vi "RX-SIS-BPCS-Modbus (SubVI).vi"(8 "error in (no error)":errorcluster, 11 "Modbus Master in":refnum<class "Modbus Master.lvclass">) -> (0 "error out":errorcluster, 1 "SIS-10SDV501":bool, 2 "SIS-10SDV500":bool, 3 "Modbus Master out":refnum<class "Modbus Master.lvclass">, 5 "SIS-10SDV502":bool, 7 "SIS-BPCS-RX-Array":bool[](array[boolean]))   [LabVIEW 2018]
uses:
  <vilib>/Modbus/master/Modbus Master.lvclass
  BPCS Global Variables.vi
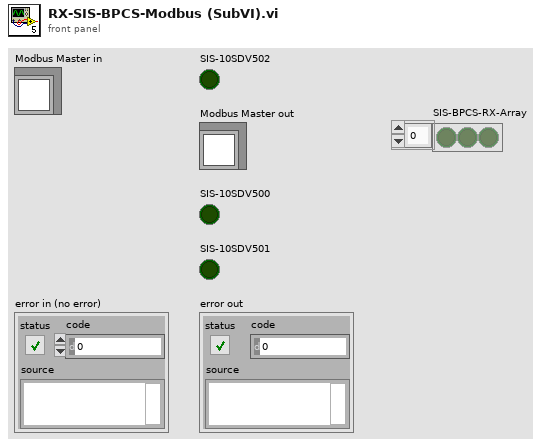
[diagram p1: front panel]
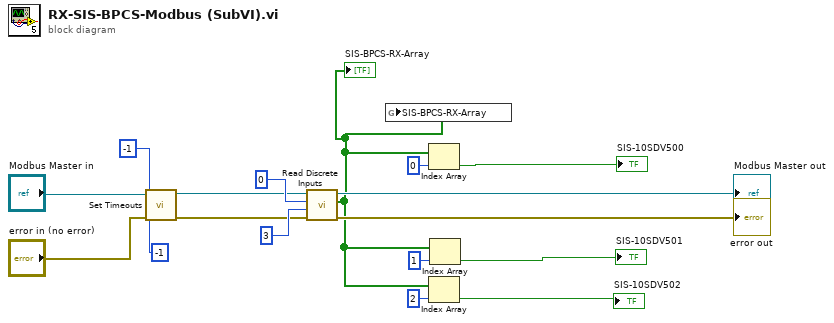
[diagram p0: block diagram]
diagram:
  n1 = call <vilib>:"Set Timeouts.vi"("error in (no error)"="error in (no error)", "write operation timeout (ms)"=-1, "read operation timeout (ms)"=-1, "Modbus master in"="Modbus Master in") -> ("error out"=w4:errorcluster, "Modbus master out"=w5:refnum<class "Modbus Master.lvclass">)  [unwired: 6 in]
  n2 = call-dynamic "Read Discrete Inputs.vi"("error in (no error)"=w4, "number of discrete inputs"=u16 3, "starting address"=u16 0, "Modbus master in"=w5) -> ("error out"=→"error out":errorcluster, "discrete input values"=w6:bool[], "Modbus master out"=→"Modbus Master out":refnum<class "Modbus Master.lvclass">)  [unwired: 5 in]
  "SIS-BPCS-RX-Array" <- w6
  n3 = global write "BPCS Global Variables.vi" "SIS-BPCS-RX-Array"(w6) -> ()
  n4 = Index Array(array=w6, index=0) -> (element=→"SIS-10SDV500":bool)
  n5 = Index Array(array=w6, index=2) -> (element=→"SIS-10SDV502":bool)
  n6 = Index Array(array=w6, index=1) -> (element=→"SIS-10SDV501":bool)
